vi "item selection selection force locks.vi"(8 "error in (no error)":errorcluster, 10 "Lock States":bool[](array[boolean]), 11 "Loop data":T1) -> (0 "error out":errorcluster, 3 "Loop data":T1)   [LabVIEW 2020, in "UI_ItemSelect.lvlib"]
uses:
  UI_ItemSelect.lvlib
  Tree item select loop data.ctl
  Item select ref type.ctl
  Tree item loop data.ctl
  Tree item selection indices.ctl
  checkbox state.ctl
  item select tree lock states.ctl
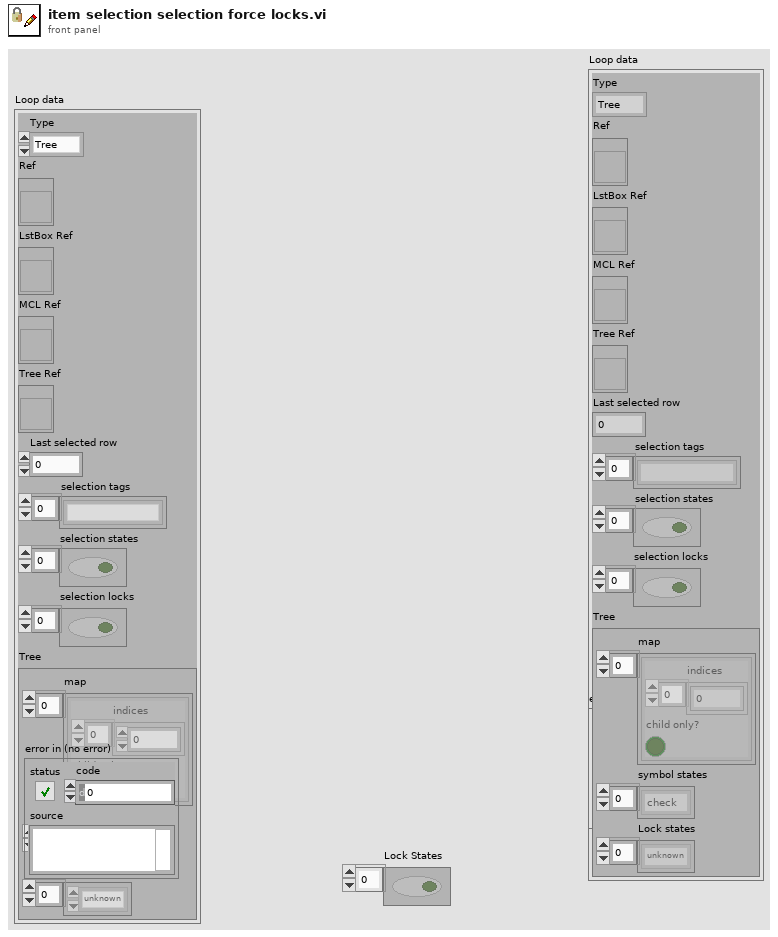
[diagram p1: front panel]
types:
  T1 = typedef "UI_ItemSelect.lvlib/Tree item select loop data.ctl" = cluster{"Type":T2, "Ref":refnum<vi>, "LstBox Ref":refnum<vi>, "MCL Ref":refnum<vi>, "Tree Ref":refnum<vi>, "Last selected row":i32, "selection tags":string[], "selection states":bool[], "selection locks":bool[], "Tree":T3}
  T2 = typedef "UI_ItemSelect.lvlib/Item select ref type.ctl" = enum16{"Tree", "MCL", "ListBox"}
  T3 = typedef "UI_ItemSelect.lvlib/Tree item loop data.ctl" = cluster{"map":T4[], "symbol states":T5[], "Lock states":T6[]}
  T4 = typedef "UI_ItemSelect.lvlib/Tree item selection indices.ctl" = cluster{"indices":i32[], "child only?":bool}
  T5 = typedef "UI_ItemSelect.lvlib/checkbox state.ctl" = enum16{"unknown", "check", "some", "no check"}
  T6 = typedef "UI_ItemSelect.lvlib/item select tree lock states.ctl" = enum16{"unknown", "locked", "unlocked"}
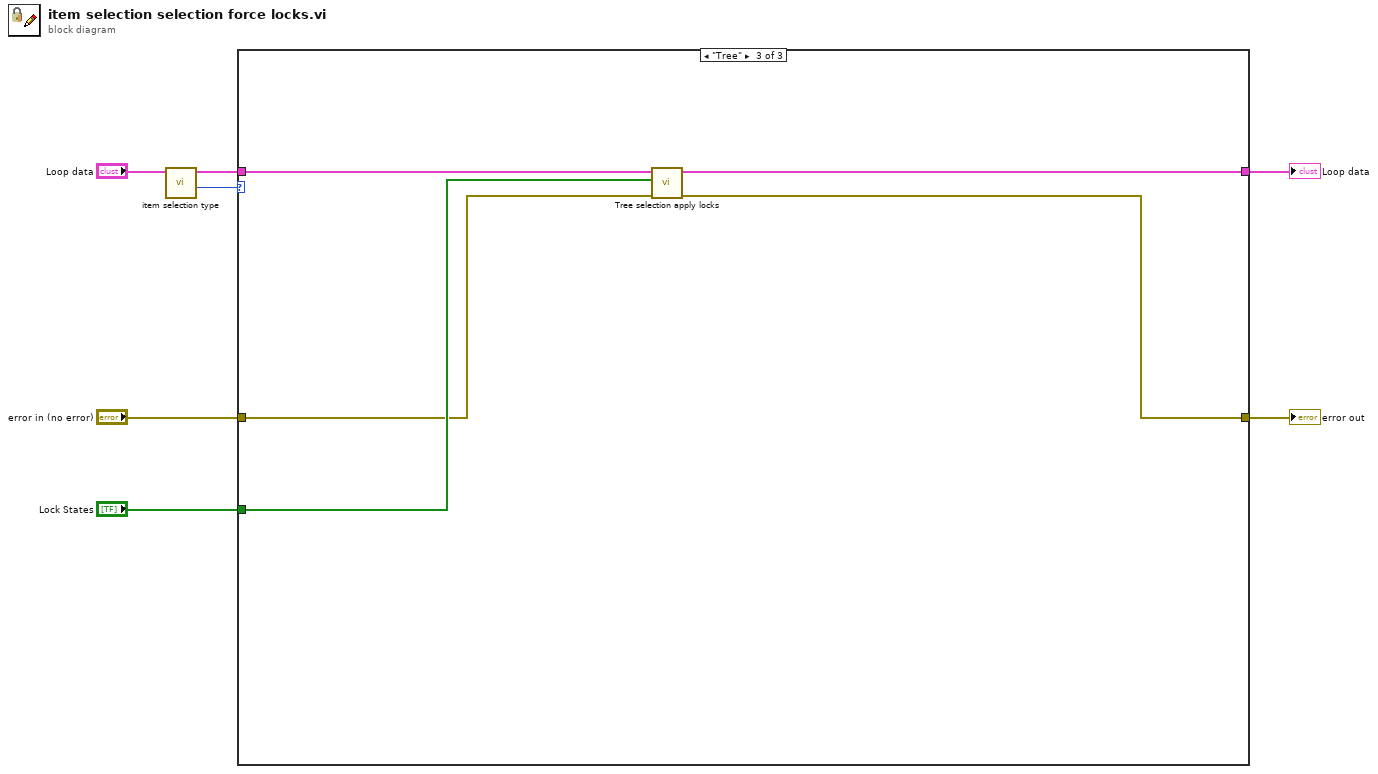
[diagram p0: block diagram]
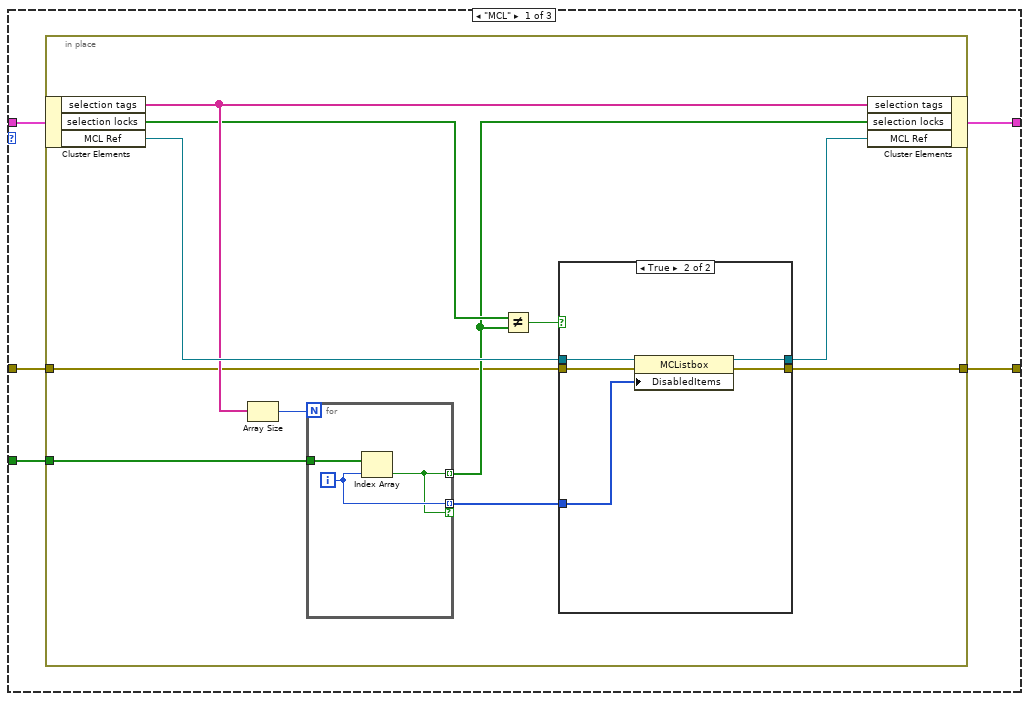
[diagram p2: hidden frame]
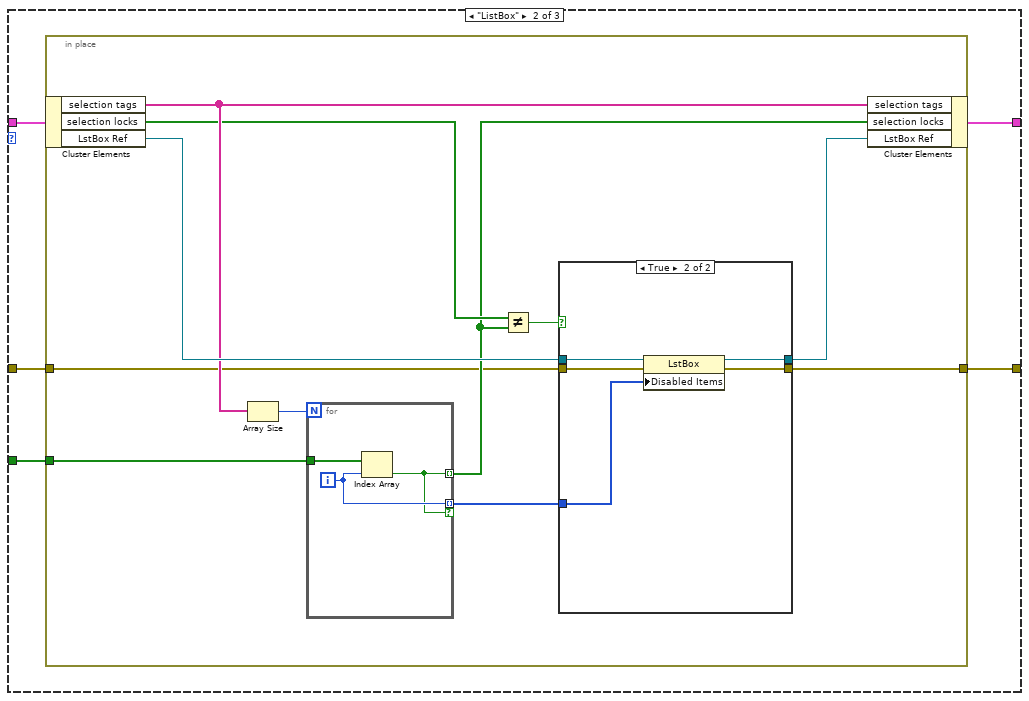
[diagram p4: hidden frame]
diagram:
  n1 = call "item selection type.vi"("Loop data"="Loop data") -> ("Type"=w4:T2, "Loop data"=w5:T1)  [unwired: 9 in]
  n2 = case shown="\"Tree\"" w4 {
    tunnel: "Lock States" -> [w12 w38 w62]
    tunnel: w5 -> [w11 w37 w64]
    tunnel: "error in (no error)" -> [w10 w36 w61]
    tunnel: [w9 w35 w60] -> w2
    tunnel: [w8 w34 w63] -> w1
    frame "MCL" {
      n3 = in-place {
        in-place-border: w12 -> [w20]
        in-place-border: w10 -> [w16]
        in-place-border: [w14] -> w9
        n4 = in-place-cluster #1(w11) -> ("selection tags"=w22:string[], "selection locks"=w19:bool[], "MCL Ref"=w23:refnum<vi>)
        n5 = Array Size(array=w22) -> (size(s)=w21:i32)
        n6 = for {
          N: w21 -> [_]
          tunnel: w20 -> [w26]
          tunnel: [w24] -> w18 mode=indexing
          tunnel: [w25] -> w13 mode=indexing if=w24
          i -> [w25]
          n7 = Index Array(array=w26, index=w25) -> (element=w24:bool)
        }
        n8 = Not Equal?(x=w19, y=w18) -> (x != y?=w17:bool)
        n9 = case shown="True" w17 {
          tunnel: w23 -> [w28 w33]
          tunnel: w16 -> [w27 w32]
          tunnel: [w28 w31] -> w15
          tunnel: [w27 w30] -> w14
          tunnel: w13 -> [_ w29]
          frame False {
          }
          frame True {
            n10 = property class="MCListbox"(reference=w33, error in=w32, "DisabledItems"=w29) -> (reference out=w31:refnum<vi>, error out=w30:errorcluster)
          }
        }
        n11 = in-place-cluster #1("selection tags"=w22, "selection locks"=w18, "MCL Ref"=w15) -> (w8:T1)
      }
    }
    frame "ListBox" {
      n12 = in-place {
        in-place-border: w38 -> [w46]
        in-place-border: w36 -> [w42]
        in-place-border: [w40] -> w35
        n13 = in-place-cluster #2(w37) -> ("selection tags"=w48:string[], "selection locks"=w45:bool[], "LstBox Ref"=w49:refnum<vi>)
        n14 = Array Size(array=w48) -> (size(s)=w47:i32)
        n15 = for {
          N: w47 -> [_]
          tunnel: w46 -> [w52]
          tunnel: [w50] -> w44 mode=indexing
          tunnel: [w51] -> w39 mode=indexing if=w50
          i -> [w51]
          n16 = Index Array(array=w52, index=w51) -> (element=w50:bool)
        }
        n17 = Not Equal?(x=w45, y=w44) -> (x != y?=w43:bool)
        n18 = case shown="True" w43 {
          tunnel: w49 -> [w54 w59]
          tunnel: w42 -> [w53 w58]
          tunnel: [w54 w57] -> w41
          tunnel: [w53 w56] -> w40
          tunnel: w39 -> [_ w55]
          frame False {
          }
          frame True {
            n19 = property class="LstBox"(reference=w59, error in=w58, "Disabled Items"=w55) -> (reference out=w57:refnum<vi>, error out=w56:errorcluster)
          }
        }
        n20 = in-place-cluster #2("selection tags"=w48, "selection locks"=w44, "LstBox Ref"=w41) -> (w34:T1)
      }
    }
    frame "Tree" {
      n21 = call "Tree selection apply locks.vi"("error in (no error)"=w61, "Lock States"=w62, "Loop data"=w64) -> ("error out"=w60:errorcluster, "Loop data"=w63:T1)  [unwired: 7 in]
    }
  }
  "error out" <- w2
  "Loop data" <- w1
